vi "sequence simple.vi"() -> ()   [LabVIEW 2013]
uses:
  result/result.lvclass
  standard action/wait action/wait action.lvclass
  result/result.lvclass/result.ctl
  result/get data.vi
  result/get error.vi
  result/get generating action.vi
  result/get owning task.vi
  result/get subresults.vi
  dispatcher/thread pool.lvclass
  standard reporters/event reporter/event reporter.lvclass
  standard tasks/sequence task/sequence task.lvclass
panel:
  out "owning task":string
  out "generating action":string
  out "error":errorcluster
  out "data":variant
  out "accessors:subresults":refnum<class "result.lvclass">[][](array[class])
  out "Array 4":string[](array[string])
  out "Array 3":string[](array[string])
  out "Array 2":errorcluster[](array[cluster])
  out "Array":variant[](array[variant])
  out "Time":u32
  out "result":refnum<class "result.lvclass">
  out "error out":errorcluster
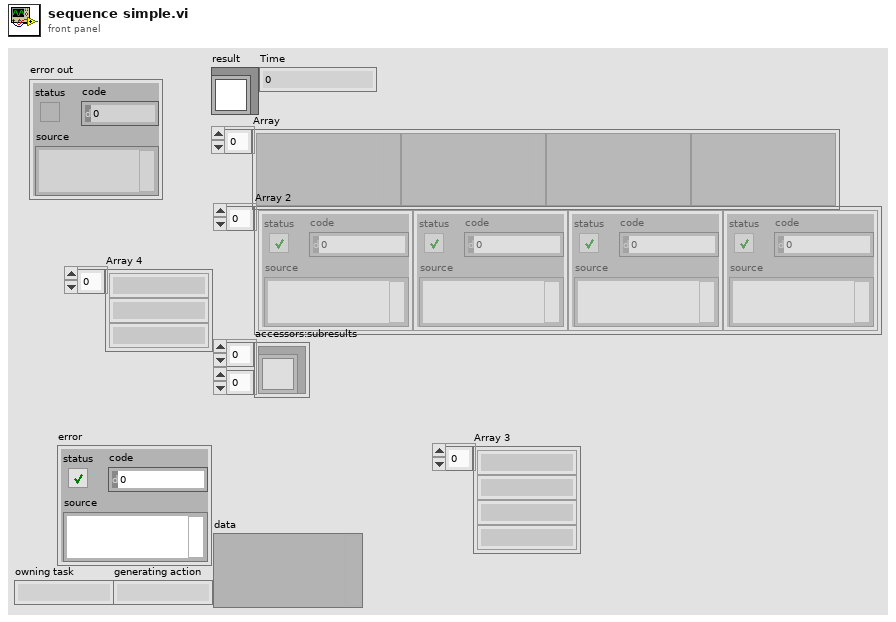
[diagram p1: front panel]
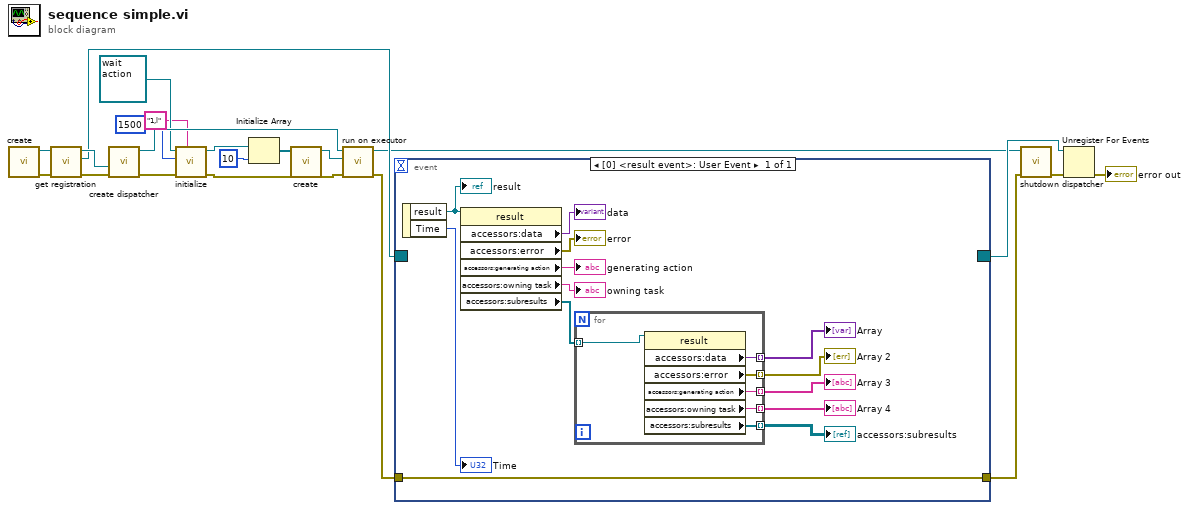
[diagram p0: block diagram]
diagram:
  n1 = call "create.vi"() -> ("error out"=w16:errorcluster, "event reporter out"=w17:refnum<class "event reporter.lvclass">)  [unwired: 10 in]
  n2 = call "get registration.vi"("error in"=w16, "event reporter in"=w17) -> ("error out"=w14:errorcluster, "result registration"=w13:refnum<event-registration>, "event reporter out"=w15:refnum<class "event reporter.lvclass">)  [unwired: 7 in]
  n3 = call "create dispatcher.vi"("error in"=w14, "default reporter"=w15) -> ("error out"=w19:errorcluster, "dispatcher"=w21:refnum<data-value>)  [unwired: 8 in]
  n4 = call-dynamic "initialize.vi"("action name"="1,l", "error in"=w19, "parameters"=1500, "action in"=refnum<class "wait action.lvclass"> refnum ("wait action.lvclass")) -> ("error out"=w2:errorcluster, "action out"=w6:refnum<class "wait action.lvclass">)  [unwired: 6 in]
  n5 = Initialize Array(w6, 10 ("dimension size")) -> (w4:refnum<class "wait action.lvclass">[])
  n6 = call "create.vi"("actions"=w4) -> ("sequence task out"=w3:refnum<class "sequence task.lvclass">)  [unwired: 10 in]
  n7 = call "run on executor.vi"("error in"=w2, "task"=w3, "dispatcher"=w21) -> ("error out"=w7:errorcluster, "dispatcher out"=w11:refnum<data-value>)  [unwired: 7 in]
  n8 = event shown="[0] <result event>: User Event" {
    selector: w13 -> [_]
    dyn-events: [_] -> w12
    timeout: _ -> [_]
    tunnel: [w33] -> w8
    tunnel: w7 -> [w33]
    event User Event {
      n9 = event-data() -> ("result"=w32:refnum<class "result.lvclass">, "Time"=→"Time":u32)  [unwired: 1 in]
      "result" <- w32
      n10 = property class="result"(reference=w32) -> ("accessors:data"=→"data":variant, "accessors:error"=→"error":errorcluster, "accessors:generating action"=→"generating action":string, "accessors:owning task"=→"owning task":string, "accessors:subresults"=w31:refnum<class "result.lvclass">[])  [unwired: 1 in, 2 out]
      n11 = for {
        tunnel: w31 -> [w40] mode=indexing
        tunnel: [w39] -> w30 mode=indexing
        tunnel: [w38] -> w29 mode=indexing
        tunnel: [w37] -> w28 mode=indexing
        tunnel: [w36] -> w27 mode=indexing
        tunnel: [w35] -> w26 mode=indexing
        n12 = property class="result"(reference=w40) -> ("accessors:data"=w39:variant, "accessors:error"=w38:errorcluster, "accessors:generating action"=w37:string, "accessors:owning task"=w36:string, "accessors:subresults"=w35:refnum<class "result.lvclass">[])  [unwired: 1 in, 2 out]
      }
      "Array" <- w30
      "Array 2" <- w29
      "Array 3" <- w28
      "Array 4" <- w27
      "accessors:subresults" <- w26
    }
  }
  n13 = call "shutdown dispatcher.vi"("error in"=w8, "dispatcher"=w11) -> ("error out"=w10:errorcluster)  [unwired: 9 in]
  n14 = Unregister For Events(event registration refnum=w12, error in=w10) -> (error out=→"error out":errorcluster)
